vi "AlliGator Global Fit Decays.vi"(6 "IRF":cluster{"t Array":dbl[], "IRF Array":dbl[]}, 8 "error in (no error)":errorcluster, 10 "Abort Fit":refnum<vi>, 11 "Decay Graph":refnum<vi>) -> (0 "Error Out":errorcluster, 1 "Reduced Chi^2":dbl, 2 "R^2":dbl, 3 "Best Fit Parameters":dbl[](array[numeric]), 4 "Fit Output Message":string, 5 "Aborted?":bool)   [LabVIEW 2021, in "AlliGator Global Decay Fit.lvlib"]
uses:
  AlliGator Global Decay Fit.lvlib
  Settings/AlliGator Settings.lvlib
  Settings/AlliGator Settings List.ctl
  Fits/Decay Convolution/Decay Model.ctl
  Fits/Fits.lvlib
  Fits/Residual Type.ctl
  Fits/IRF(X)PSED/Decay Fit Parameters In List.ctl
  Decay Fit/AlliGator Decay Fit Parameter Constraints 2.ctl
  Decay Fit/AlliGator Decay Fit.lvlib
  Graphs/XY Graph/XY Graph Add-Ons.lvlib
  Fits/Global Fits/Global Fit Parameters Information.ctl
  Fits/Global Fits/Global Fit Data.ctl
  Time/Time.lvlib
  Fits/Abort Fit Global.vi
  Globals, Variables, Constants/AlliGator Globals, Variables & Constants.lvlib
  Globals, Variables, Constants/AlliGator Variables List.ctl
  Fits/Fit Calculation Method.ctl
  Fits/Non-linear Fitting Algorithm.ctl
  Fits/Non-linear Fitting Method v2.ctl
  Fits/Optimal Offset Selection Criterion.ctl
  Graphs/XY Graph/XY Graph Add Multiplots with Names v2.vi
  Graphs/LabVIEW Plot Interpolation.ctl
  Graphs/Graphs.lvlib
  Fits/IRF(X)PSED/Fit Weights Type v2.ctl
  Fits/IRF(X)PSED/Decay Fit Options v4.ctl
panel:
  # "see the License on the block diagram (Ctrl+E or Window:Show Block Diagram)"
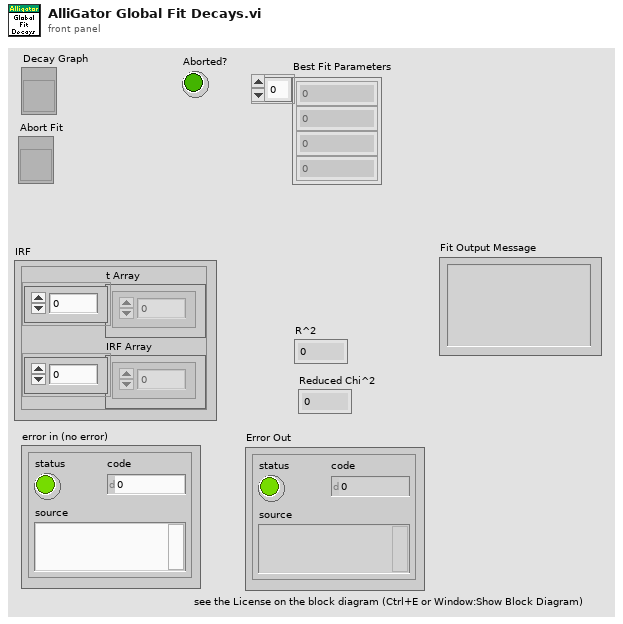
[diagram p1: front panel]
types:
  T1 = typedef "Fits.lvlib/Optimal Offset Selection Criterion.ctl" = enum16{"Min Chi^2", "Max R^2"}
  T2 = typedef "AlliGator Settings.lvlib/AlliGator Settings List.ctl" = enum16{"GUI:Visible Settings Tab", "GUI:Last Run Version", "Source Image:Use Image Histogram for Contrast", "Source Image:Low Count Pixels Rejection Options", "Source Image:High Count Pixels Rejection Options", "Source Image:Use Image Brightness", "Source Image:Blend Overlay with Image Background", "Source Image:Use Fixed ROI Diameter", "Source Image:ROI Diameter", "Source Image:ROI Center Color", "Source Image:Peak Threshold", "Source Image:Intensity Threshold", "Source Image:Image Binning Options", "Source Image:Image Smoothing Options", "Source Image:Image Histogram Active", "Source Image:Invert Binary Mask", "Source Image:Hot Pixel Removal", "Source Image:Overlay Analyzed ROI Center", "Source Image:Auto-Adjust Contrast", "Source Image:Histogram Lower Percentile", "Source Image:Histogram Upper Percentile", "Source Image:Save Source Image", "Source Image:Scale Bar Options", "Source Image:Image Resolution (Pixel Size)", "Source Image:Flatfield Correction", "Source Image:Show Dead Left Columns Correction", "Source Image:Dead Left Columns Correction", "Source Image:Image Pre-Processing Operations Order", "Source Image:Overlay ROI Median", "Source Image:Median Overlay Color", "Data Information:Gate Width", "Data Information:Nanotime Gate Separation", "Data Information:Macrotime Gate Separation", "Data Information:Gate Step", "Data Information:# Gates", "Data Information:Gate Image Exposure", "Data Information:Gate Image Integration", "Data Information:Gates to Skip", "Data Information:Gates to Keep", "Data Information:Define Gates to", "Data Information:Channel Name", "Data Information:Available Channel Names", "Data Information:Channel Arithmetic", "Data Information:Background File Subtraction", "Data Information:Background File", "Data Information:Background Scaling Factor", "Data Information:Background Pile-up Correction", "Data Information:Background Pixel Well Capacity", "Data Information:Laser Period", "Data Information:SYNC Period", "Data Information:Pile-up Correction", "Data Information:Pixel Well Capacity", "Data Information:Dataset Scaling Factor", "Fluorescence Decay_Decay Pre-Processing:Reverse Gates", "Fluorescence Decay_Decay Pre-Processing:Verbose Decay Pre-Processing", "Fluorescence Decay_Decay Pre-Processing:Use Decay Pre-Processing", "Fluorescence Decay_Decay Pre-Processing:Background Subtraction", "Fluorescence Decay_Decay Pre-Processing:Background Definition Range", "Fluorescence Decay_Decay Pre-Processing:Baseline Subtraction Method", "Fluorescence Decay_Decay Pre-Processing:Decay Pre-Processing Operations Order", "Fluorescence Decay_Decay Pre-Processing:Smoothing Parameter", "Fluorescence Decay_Decay Pre-Processing:Shift Decay", "Fluorescence Decay_Decay Pre-Processing:Decay Shift Parameters", "Fluorescence Decay_Decay Pre-Processing:Fold Decay", "Fluorescence Decay_Decay Pre-Processing:# Folds", "Fluorescence Decay_Decay Pre-Processing:1-Normalize Decay", "Fluorescence Decay_Decay Pre-Processing:[0-1]-Normalize Decay", "Fluorescence Decay_Decay Pre-Processing:Smoothen Decay", "Fluorescence Decay_Decay Pre-Processing:Extrapolate Decay", "Fluorescence Decay_Decay Pre-Processing:Use Periodicity", "Fluorescence Decay_Decay Pre-Processing:Use Cursors", "Fluorescence Decay_Decay Pre-Processing:Tail Fraction", "Fluorescence Decay_Decay Pre-Processing:Head Fraction", "Fluorescence Decay_Decay Pre-Processing:Additional Points", "Fluorescence Decay_Decay Pre-Processing:Straighten Decay", "Fluorescence Decay_Decay Pre-Processing:Constant Background", "Fluorescence Decay_Decay Pre-Processing:Pixel-Normalize Decay", "Fluorescence Decay_Advanced Analysis:Extract IRF instead of Decay", "Fluorescence Decay_Advanced Analysis:IRF Extraction Options", "Fluorescence Decay_Advanced Analysis:IRF Optimization Options", "Fluorescence Decay_Advanced Analysis:Square Pulse Options", "Fluorescence Decay_Advanced Analysis:IRF Order", "Fluorescence Decay_Advanced Analysis:IRF Time Constants", "Fluorescence Decay_Advanced Analysis:Wavelet Analysis Options", "Fluorescence Decay_Advanced Analysis:Average Lifetime Options", "Fluorescence Decay_Fit Options:Fit Options", "Fluorescence Decay_Fit Options:Use Legacy Fitting Approach", "Fluorescence Decay_Fit Options:Use Data Information Laser Period", "Fluorescence Decay_Fit Parameters:Displayed Fit Parameters", "Fluorescence Decay_Fit Parameters:Fit Parameter Constraints", "Fluorescence Decay_Fit Parameters:Export Tabulated Results", "Fluorescence Decay_Fit Parameters:MLE Baseline Offset Type", "Fluorescence Decay_Fit Parameters:MLE Baseline Offset", "Fluorescence Decay_Fit Parameters:Guess Parameter Names", "Fluorescence Decay_Fit Parameters:Guess Parameter Values", "Fluorescence Decay_Fit Parameters:Guess Parameters Options", "Fluorescence Decay_Fit Parameters:Optimal Offset Selection Criterion", "Fluorescence Decay_Styles:Show Last Decay Only", "Fluorescence Decay_Styles:Decay Graph Color Array", "Fluorescence Decay:Decay Graph Active", "Fluorescence Decay Statistics:Min Peak Value", "Fluorescence Decay Statistics:Reject Low Decay Peak Pixels", "Fluorescence Decay Statistics:Reject High Decay Peak Pixels", "Fluorescence Decay Statistics:Max Peak Value", "Time Traces:Use File Timestamp", "Time Traces:Time Step", "Time Traces:Use Intensity Correction File", "Time Traces:Intensity Correction File", "Phasor Plot:Phasor Plot Smoothing Options", "Phasor Plot:Phasor Plot Size", "Phasor Plot:Phasor Plot Graphics Options", "Phasor Plot:Cumulative Phasor Plot", "Phasor Plot:Use Phasor Brightness", "Phasor Plot:Blend Overlay with Phasor Background", "Phasor Plot:Save Phasor Plot", "Phasor Plot:Show References", "Phasor Plot:Phasor Ratio Decay Range", "Phasor Plot:Exponential Fading", "Phasor Plot:Phasor Ratio Reference Colors", "Phasor Plot:Reference Radius", "Phasor Plot:Show Color Map Vertices", "Phasor Plot:Phasor Plot Active", "Phasor Plot:Phasor Ratio Color Map Type", "Phasor Plot:Phasor Ratio Color Map", "Phasor Plot:Phasor Ratio Display Range", "Phasor Plot:Selected Image ROI(s)", "Phasor Plot:All Image ROIs", "Phasor Plot:Selected Phasor Plot ROI(s)", "Phasor Plot:All Phasor Plot ROIs", "Phasor Plot:Phasor Ratio Color-Coded Quantity", "Phasor Plot:Store Phasor Harmonics", "Phasor Plot:Draw Reference Segment", "Phasor Plot:User-Defined Quantity", "Phasor Plot:Color Scale High Color", "Phasor Plot:Color Scale Low Color", "Phasor Plot:Intensity-weighted Phasor Plot", "Phasor Graph:Phasor Frequency", "Phasor Graph:Phasor Ratio Type", "Phasor Graph:Pixel-level Phasor Computation", "Phasor Graph:Save Phasor Graph", "Phasor Graph:Phasor Graph Active", "Phasor Graph:Phasor SDV Options", "Phasor Graph:Intensity-weighted Phasor Graph", "Phasor Graph:Define Shortest Lifetime as", "Phasor Calibration:Use Backup Calibration if needed", "Phasor Calibration:Backup Calibration Type", "Phasor Calibration:Calibration Type", "Phasor Calibration:Calibration Lifetime", "Phasor Calibration:Calibration Map Algorithm", "Single-Exponential Phasor Locus (SEPL):Gate Parameters", "Single-Exponential Phasor Locus (SEPL):User-defined Gate", "Single-Exponential Phasor Locus (SEPL):User-defined IRF", "Single-Exponential Phasor Locus (SEPL):Phasor Parameters", "Single-Exponential Phasor Locus (SEPL):Decay & IRF Parameters", "Single-Exponential Phasor Locus (SEPL):Display Parameters", "Lifetime Analysis:Decay Analysis Parameters", "Lifetime Analysis:Lifetime Map Active", "Plugins:Python Settings", "Miscellaneous:Verbose Mode", "Miscellaneous:Beep after Script", "Miscellaneous:Saved Image File Format", "Miscellaneous:Exported Gate Image Settings", "Miscellaneous:Include Loading in Timing", "Miscellaneous:Verbose Settings Mode", "Miscellaneous:Histogram Options", "Miscellaneous:Beep on Error", "Miscellaneous:# Logical Processors Used", "Miscellaneous:ROI Description Max Characters", "Miscellaneous:Verbose Error Mode", "Miscellaneous:Transparent Mask Color"}
  T3 = typedef "Fits.lvlib/Decay Fit Options v4.ctl" = cluster{"Show Fit Residuals":bool, "Fit Model":T4, "Residual Type":T5, "Max Decay Percentile":dbl, "Min Decay Percentile":dbl, "Show Full Decay":bool, "Weights":T6, "Fitting Method":T7, "Compute Parameter Uncertainties":bool, "Periodic Boundaries":bool, "Model Calculation":T8, "Period":dbl[unit], "Termination Criteria":cluster{"Max Iterations":i32, "Max Function Calls":i32, "Max Time":dbl[unit], "Function Tolerance":dbl, "Parameter Tolerance":dbl, "Gradient Tolerance":dbl, "Min Lambda":dbl, "Max Lambda":dbl, "Initial Tick Count":u32}, "Offset Resolution":dbl[unit], "Use Local IRF":bool, "Fitting Algorithm":T9, "Show Confidence Interval ":bool, "Confidence Level":dbl}
  T4 = typedef "Fits.lvlib/Decay Model.ctl" = enum16{"1-Exponential", "2-Exponentials"}
  T5 = typedef "Fits.lvlib/Residual Type.ctl" = enum16{"Standard", "Normalized", "Reduced"}
  T6 = typedef "Fits.lvlib/Fit Weights Type v2.ctl" = enum16{"Unweighted", "1/Variance (Neyman)", "1/Variance (Pearson)", "Best of All"}
  T7 = typedef "Fits.lvlib/Non-linear Fitting Method v2.ctl" = enum16{"Least Square", "Least Absolute Residual", "Bisquare", "MLE", "-", "Best of All"}
  T8 = typedef "Fits.lvlib/Fit Calculation Method.ctl" = enum16{"Simulation", "Convolution", "Integration"}
  T9 = typedef "Fits.lvlib/Non-linear Fitting Algorithm.ctl" = enum16{"Levenberg-Marquardt", "Trust-Region Dogleg"}
  T10 = cluster{"Max Iterations":i32, "Max Function Calls":i32, "Max Time":dbl[unit], "Function Tolerance":dbl, "Parameter Tolerance":dbl, "Gradient Tolerance":dbl, "Min Lambda":dbl, "Max Lambda":dbl, "Initial Tick Count":u32}
  T11 = typedef "XY Graph Add-Ons.lvlib/XY Graph Refnum.ctl" = refnum<vi>
  T12 = typedef "AlliGator Globals, Variables & Constants.lvlib/AlliGator Variables List.ctl" = enum16{"---- GUI ----", "GUI:Initialization Status", "GUI:State Indicators Refnum", "GUI:Original AlliGator Menu Items", "GUI:Current Action Loop State", "GUI:Script in progress", "GUI:Playback", "GUI:Loop Playback", "GUI:Search ROI Used", "GUI:Search ROI", "Decay Graph Max Legend Size", "Intensity Graph Max Legend Size", "Decay Statistics Graph Max Legend Size", "Phasor Graph Max Legend Size", "Phasor Ratio Graph Max Legend Size", "Lifetime Graph Max Legend Size", "---- Files ----", "Files:Export Dataset Frames as Individual Files", "Files:Show Batch Export Help Balloons", "Files:Frames in Dataset", "Files:ptu File Frame Start Indices", "Files:Current Frame in Dataset", "Files:Current Frame Timestamp", "Files:Dataset Loaded", "Files:Dataset Metadata", "Files:Dataset Channel", "Files:Dataset Data Description", "Files:Background Dataset Metadata", "Files:Background Dataset Channel", "Files:Background Dataset Data Description", "Files:Background File Subtraction", "Files:Background File Path", "Files:Background File Pile-up Correction", "Files:Background File Pixel Well Capacity", "Files:Background File Scaling Factor", "Files:Current Dataset Load Settings", "Files:Dataset Path", "Files:ICCD-specific Information", "Files:Macrotime Gate Separation", "------ Python Plugins ------", "Python Plugins:Information", "Python Plugins:Python Session", "Python Plugins:Valid Python Session?", "---- Source Image ----", "Source Image:ROIs", "Source Image:Current ROI", "Source Image:ROI Event Refnum", "X_Source Image:Display Range", "X_Source Image:Palette Information", "X_Source Image:Type of Displayed Image", "X_Time Gate Slider", "Source Image:Palette List", "Source Image:Scale", "Source Image:ROI Overlay Color", "Source Image:Overlay to Erase", "Source Image:Is Displayed Image Accumulated", "Source Image:White Light Image Modified", "Source Image:Mask Image Modified", "---- Image Profile Window ----", "Image Profile:Window Event Refnum", "Image Profile:IntensityType", "Image Profile:Intensity Average Type", "Image Profile:Intensity-weighted SDV", "Image Profile:Box Profile Type", "Image Profile:Window Open", "Image Profile:Plotted Fit Parameter", "------ Phasor Graph -------", "Phasor Graph:Show Line", "---- Phasor Plot ---", "Phasor Plot:Parameters Changed", "Phasor Plot:FLI Dataset Modified since last Calculation", "Phasor Harmonics Data", "Selected Phasor Harmonics", "Phasor Harmonic Manager Event Refnum", "Phasor Plot:ROIs", "Phasor Plot:Current ROI", "Phasor Plot:ROI Event Refnum", "Phasor Plot:Image Reference Points", "Phasor Plot:Computed", "Phasor Plot:Palette Information", "Phasor Plot:Palette List", "Phasor Plot:Phasor Ratio Palette Information", "Phasor Plot:Phasor Ratio Palette List", "Phasor Plot:Image Scale", "Phasor Plot:Image Overlay to Erase", "Phasor Plot:Image Elements to Update", "Phasor Plot:Current Calculation Parameters", "Phasor Plot:Current Calibration Options", "Phasor Plot:Reset Cumulated Phasor Plot", "Phasor Plot:Reference 1", "Phasor Plot:Lifetime Reference 1", "Phasor Plot:Reference 1 Frequency", "Phasor Plot:Reference 2", "Phasor Plot:Lifetime Reference 2", "Phasor Plot:Reference 2 Frequency", "---- Decay Analysis ----", "Number of Selected Decays to Fit", "LS Fit Results", "LAR Fit Results", "BS Fit Results", "Last Decay Max - Min", "Best Fit Parameters", "Best Fit Parameter Names", "Actual Size X", "Actual Size Y", "Binning X", "Binning Y", "Actual # Gates", "Dataset Number", "Gates to...", "Gates Skipped", "Gates to keep", "Gate Step", "Gate Separation", "Reversed Gates", "Pile-up Correction", "Pixel Well Capacity", "Background Subtracted", "Background Subtraction Method", "Background Definition Range", "Background File (deprecated)", "Number of Dataset Accumulated", "Array of Accumulated Dataset Paths", "Do Averaged Datasets", "Destination File Path", "Process Plot Target", "Use 1/D as Phasor Frequency", "---- Decay Fit Parameter Map -----", "Decay Fit Parameter Map:Palette Information", "Decay Fit Parameter Map:Palette List", "Decay Fit Parameter Map:X Resolution", "Decay Fit Parameter Map:Y Resolution", "Decay Fit Parameter Map:Use Decay Fit Result Constraints", "Decay Fit Parameter Map:Decay Fit Result Constraints", "Decay Fit Parameter Map:Decay Fit Result Constraints Applied", "---- Parameter Map ----", "Parameter Map:Palette Information", "Parameter Map:Palette List", "------- Local Decay Window ---------", "Local Decay Graph Window:Event Refnum", "Local Decay Graph Window:Use normalized IRF for convolution", "----- Miscellaneous ----", "Misc:Skippable Dialog Windows Status"}
  T13 = typedef "AlliGator Decay Fit.lvlib/AlliGator Decay Fit Parameter Constraints 2.ctl" = cluster{"Fit Parameter":T14, "Min Value":dbl, "Max Value":dbl, "Global":bool, "Used":bool}
  T14 = typedef "Fits.lvlib/Decay Fit Parameters In List.ctl" = enum16{"Offset", "Baseline", "A_1", "tau_1", "A_2", "tau_2"}
  T15 = typedef "Fits.lvlib/Global Fit Data.ctl" = cluster{"Fit Data":variant, "Global Fit Parameter Information":T16, "# Points in Plots":i32[]}
  T16 = typedef "Fits.lvlib/Global Fit Parameters Information.ctl" = cluster{"Original Parameter Indices":i32[], "# Global Parameters":i32, "# Plot Specific Parameters":i32, "Global Parameter? Array":bool[]}
  T17 = typedef "Graphs.lvlib/LabVIEW Plot Interpolation.ctl" = enum16{"Point (.)", "Stepwise Right (--.)", "Line + Point (\\. /)", "Stepwise Left (.--)", "Stepwise Centered (-.-)", "Stepwise Vertical (|.|)", "Line (-)", "Use Previous Plot's Style"}
  T18 = cluster{"parameter minimum":dbl[], "parameter maximum":dbl[]}
  T19 = typedef "Fits.lvlib/Fit Plots.ctl" = cluster{"Fitted Decay":cluster{"t Array":dbl[], "Fitted Array":dbl[]}, "Residuals":cluster{"t Array":dbl[], "Residual Array":dbl[]}, "Upper CI Plot":cluster{"t Array":dbl[], "Residual Array":dbl[]}, "Lower CI Plot":cluster{"t Array":dbl[], "Residual Array":dbl[]}}
  T20 = typedef "Fits.lvlib/Non-linear Fit Output v4.ctl" = cluster{"best nonlinear fit":dbl[], "best fit parameters":dbl[], "R^2":dbl, "RMSE":dbl, "error out":errorcluster, "Fitting Method":T21, "number of function calls":i32, "number of iterations":i32, "covariance":T22, "Chi 2":dbl, "DOF":i32, "Fit Convergence Criterion":T23, "Fitting Algorithm":T9, "Weighted Fit":T6, "Gradient":dbl, "|Delta Chi 2|":dbl, "|Delta Chi 2|/Chi 2":dbl, "Max |Delta a| /|a|":dbl, "Lambda":dbl, "RSS":dbl, "AIC":dbl, "BIC":dbl, "Max number of function calls":i32, "Max number of iterations":i32, "IRF":T24, "IRF Normalization Factor":dbl, "Decay Normalization Factor":dbl, "Number of offset fits":i32, "Weighted Chi2":dbl, "Unweighted Chi2":dbl}
  T21 = typedef "Fits.lvlib/Nonlinear Fit Method.ctl" = enum16{"Least Square", "Least Absolute Residual", "Bisquare", "MLE"}
  T22 = typedef "NI_Matrix.lvlib/RealMatrix.ctl" = dbl[][]
  T23 = typedef "Fits.lvlib/Convergence Criteria.ctl" = enum16{"Continue", "Tolerances Exceeded", "Max Time Exceeded", "Max Iterations Exceeded", "Max Function Evaluations Exceeded", "Scale Range Exceeded"}
  T24 = typedef "XY Graph Add-Ons.lvlib/XY Graph Plot Data.ctl" = cluster{"X Array":dbl[], "Y Array":dbl[]}
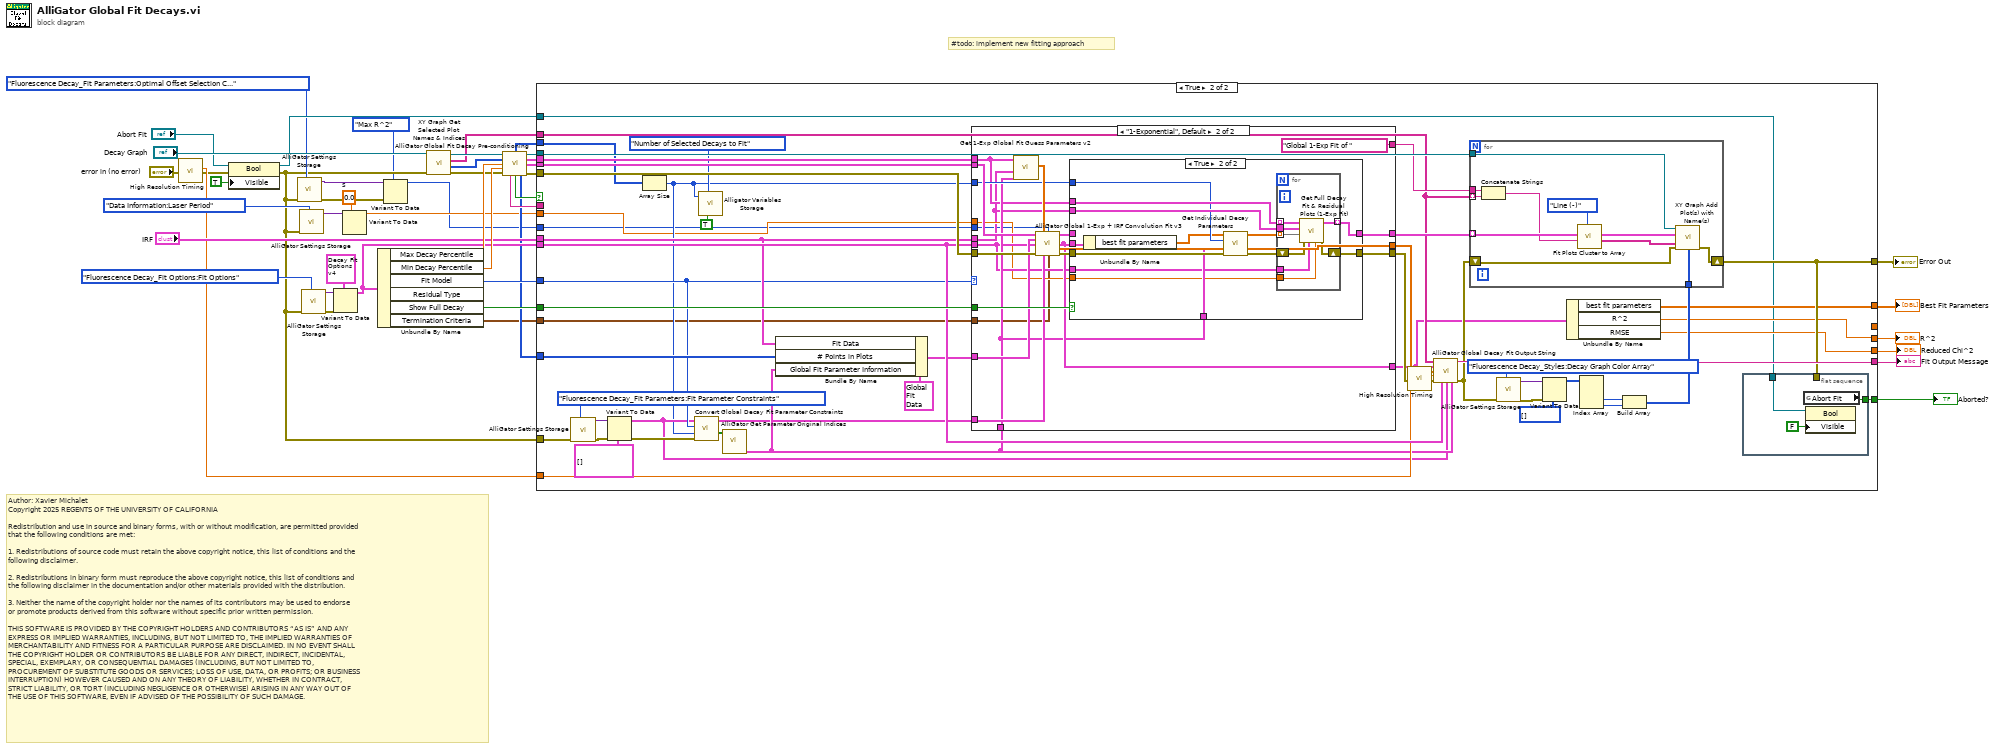
[diagram p0: block diagram]
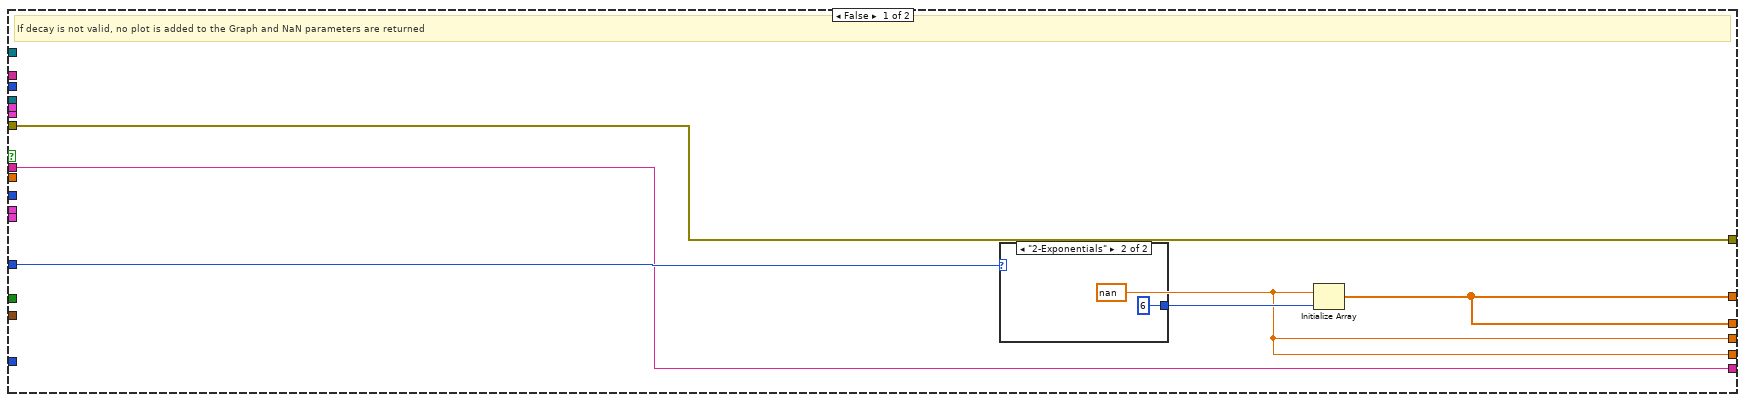
[diagram p2: hidden frame]
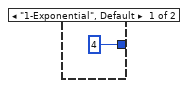
[diagram p3: hidden frame]
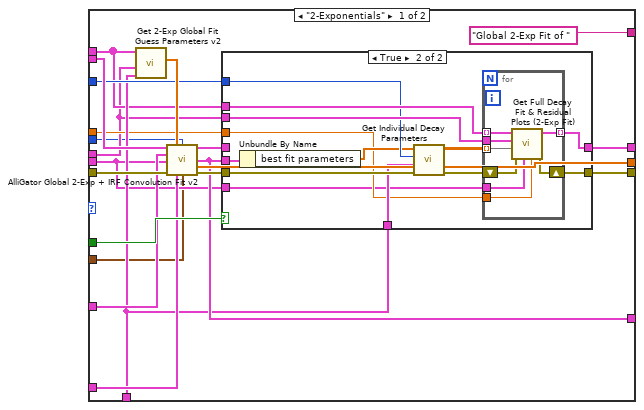
[diagram p4: hidden frame]
diagram:
  w13 = dbl[unit] 0.0  # s
  # "Author: Xavier Michalet\nCopyright 2025 REGENTS OF THE UNIVERSITY OF CALIFORNIA\n\nRedistribution and use in source and binary forms, with or without modification, are permitted provided\nthat the following conditions are met:\n\n1. Redistributions of source code must retain the above copyright notice, this list of conditions and the\nfollowing disclaimer.\n\n2. Redistributions in binary form must reproduce the above copyright notice, this list of conditions and\nthe following disclaimer in the documentation and/or other materials provided with the distribution.\n\n3. Neither the name of the copyright holder nor the names of its contributors may be used to endorse \nor promote products derived from this software without specific prior written permission.\n\nTHIS SOFTWARE IS PROVIDED BY THE COPYRIGHT HOLDERS AND CONTRIBUTORS “AS IS” AND ANY \nEXPRESS OR IMPLIED WARRANTIES, INCLUDING, BUT NOT LIMITED TO, THE IMPLIED WARRANTIES OF\nMERCHANTABILITY AND FITNESS FOR A PARTICULAR PURPOSE ARE DISCLAIMED. IN NO EVENT SHALL\nTHE COPYRIGHT HOLDER OR CONTRIBUTORS BE LIABLE FOR ANY DIRECT, INDIRECT, INCIDENTAL, \nSPECIAL, EXEMPLARY, OR CONSEQUENTIAL DAMAGES (INCLUDING, BUT NOT LIMITED TO, \nPROCUREMENT OF SUBSTITUTE GOODS OR SERVICES; LOSS OF USE, DATA, OR PROFITS; OR BUSINESS\nINTERRUPTION) HOWEVER CAUSED AND ON ANY THEORY OF LIABILITY, WHETHER IN CONTRACT, \nSTRICT LIABILITY, OR TORT (INCLUDING NEGLIGENCE OR OTHERWISE) ARISING IN ANY WAY OUT OF\nTHE USE OF THIS SOFTWARE, EVEN IF ADVISED OF THE POSSIBILITY OF SUCH DAMAGE."
  # "#todo: implement new fitting approach"
  n1 = call "High Resolution Timing.vi"("Error In"="error in (no error)") -> ("elapsed (relative) seconds"=w21:dbl, "Error Out"=w9:errorcluster)  [unwired: 16 in, 1 out]
  n2 = property class="Bool"(reference="Abort Fit", error in=w9, "Visible"=TRUE) -> (reference out=w8:refnum<vi>, error out=w5:errorcluster)
  n3 = call "AlliGator Settings Storage.vi"("AlliGator Settings List"=AlliGator_Settings_List."Fluorescence Decay_Fit Parameters:Optimal Offset Selection Criterion", "Error In"=w5) -> ("Error Out"=w4:errorcluster, "Variant Data out"=w3:variant)  [unwired: 8 in]
  n4 = call "AlliGator Settings Storage.vi"("AlliGator Settings List"=AlliGator_Settings_List."Data Information:Laser Period", "Error In"=w5) -> ("Variant Data out"=w14:variant)  [unwired: 8 in, 1 out]
  n5 = call "AlliGator Settings Storage.vi"("AlliGator Settings List"=AlliGator_Settings_List."Fluorescence Decay_Fit Options:Fit Options", "Error In"=w5) -> ("Error Out"=w41:errorcluster, "Variant Data out"=w42:variant)  [unwired: 8 in]
  n6 = Variant To Data(error in=w41, type=T3 {"Show Fit Residuals"=TRUE, "Fit Model"=enum."1-Exponential", "Residual Type"=enum."Standard", "Max Decay Percentile"=0.0, "Min Decay Percentile"=0.0, "Show Full Decay"=TRUE, "Weights"=enum."Unweighted", "Fitting Method"=enum."Least Square", "Compute Parameter Uncertainties"=TRUE, "Periodic Boundaries"=TRUE, "Model Calculation"=enum."Simulation", "Period"=1.2500000000000001e-08, "Termination Criteria"={"Max Iterations"=1000, "Max Function Calls"=0, "Max Time"=1000.0, "Function Tolerance"=1e-06, "Parameter Tolerance"=1e-06, "Gradient Tolerance"=0.0, "Min Lambda"=1e-06, "Max Lambda"=1e-06, "Initial Tick Count"=0}, "Offset Resolution"=1.2500000000000001e-08, "Use Local IRF"=TRUE, "Fitting Algorithm"=enum."Levenberg-Marquardt", "Show Confidence Interval "=TRUE, "Confidence Level"=95.0} ("Fit Options"), Variant=w42) -> (data=w32:T3)  [unwired: 1 out]
  n7 = Variant To Data(type=w13, Variant=w14) -> (data=w12:dbl[unit])  [unwired: 1 in, 1 out]
  n8 = Unbundle By Name(w32) -> ("Max Decay Percentile"=w36:dbl, "Min Decay Percentile"=w35:dbl, "Fit Model"=w31:T4, "Show Full Decay"=w34:bool, "Termination Criteria"=w11:T10)  [unwired: 1 out]
  n9 = Variant To Data(error in=w4, type=Optimal_Offset_Selection_Criterion."Max R^2" ("Optimal Offset Selection Criterion"), Variant=w3) -> (data=w1:T1)  [unwired: 1 out]
  n10 = call "XY Graph Get Selected Plot Names & Indices.vi"("error in (no error)"=w5, "XY Graph in"="Decay Graph") -> ("error out"=w17:errorcluster, "Selected Plot Indices"=w16:i32[], "Selected Plot Names"=w24:string[], "XY Graph out"=w29:T11)  [unwired: 5 in, 1 out]
  n11 = call "AlliGator Global Fit Decay Pre-conditioning.vi"("XYGraph in"=w29, "Selected Plots"=w16, "Max Decay Percentile (1)"=w36, "Min Decay Percentile (0)"=w35, "error in (no error)"=w17) -> ("Index Max Array"=w25:i32[], "XYGraph out"=w46:refnum<vi>, "Full Decays"=w23:cluster{"t Array":dbl[], "Value Array":dbl[]}[], "Clipped Decays"=w27:cluster{"t Array":dbl[], "Value Array":dbl[]}[], "Message"=w28:string, "Is Valid?"=w33:bool, "# Points"=w18:i32[], "error out"=w19:errorcluster)  [unwired: 1 in, 2 out]
  n12 = case shown="True" w33 {
    tunnel: w46 -> [_ w107]
    tunnel: [w52 w90] -> w45
    tunnel: [w47 w105] -> w44
    tunnel: [w49 w61] -> w39
    tunnel: [w49 _] -> _
    tunnel: [w48 w60] -> w38
    tunnel: w31 -> [w51 w84]
    tunnel: [w48 w59] -> w37
    tunnel: "IRF" -> [_ w88]
    tunnel: w34 -> [_ w101]
    tunnel: w19 -> [w52 w100]
    tunnel: w32 -> [_ w98]
    tunnel: w28 -> [w47 _]
    tunnel: w27 -> [_ w97]
    tunnel: w25 -> [_ w64]
    tunnel: w24 -> [_ w95]
    tunnel: w23 -> [_ w96]
    tunnel: w21 -> [_ w93]
    tunnel: [_ w91] -> w20
    tunnel: w18 -> [_ w87]
    tunnel: w5 -> [_ w78]
    tunnel: w12 -> [_ w58]
    tunnel: w11 -> [_ w57]
    tunnel: w8 -> [_ w56]
    tunnel: w1 -> [_ w55]
    frame False {
      w48 = nan ("element")
      # "If decay is not valid, no plot is added to the Graph and NaN parameters are returned"
      n13 = case shown="\"2-Exponentials\"" w51 {
        tunnel: [4 ("dimension size") 6 ("dimension size")] -> w50
        frame "1-Exponential", Default {
        }
        frame "2-Exponentials" {
        }
      }
      n14 = Initialize Array(w48, w50) -> (w49:dbl[])
    }
    frame True {
      n15 = call "AlliGator Settings Storage.vi"("AlliGator Settings List"=AlliGator_Settings_List."Fluorescence Decay_Fit Parameters:Fit Parameter Constraints", "Error In"=w78) -> ("Error Out"=w80:errorcluster, "Variant Data out"=w81:variant)  [unwired: 8 in]
      n16 = Variant To Data(error in=w80, type=T13[] [] ("Fit Parameter Constraints"), Variant=w81) -> (data=w75:T13[], error out=w76:errorcluster)
      n17 = Array Size(array=w64) -> (size(s)=w63:i32)
      n18 = call "Convert Global Decay Fit Parameter Constraints.vi"("Error In"=w76, "# Plots"=w63, "Fit Model"=w84, "Fit Parameter Constraints"=w75) -> ("Global Parameters?"=w83:bool[], "Parameter Bounds"=w82:T18)  [unwired: 5 in, 1 out]
      n19 = call "Alligator Variables Storage.vi"("Get(F)/Set"=TRUE, "AlliGator Variable"=AlliGator_Variables_List."Number of Selected Decays to Fit" ("Alligator Variable"), "Data in"=w63) -> ()  [unwired: 6 in, 3 out]
      n20 = call "AlliGator Get Parameter Original Indices.vi"("Parameter Types"=w83) -> ("Global Fit Parameter Info"=w85:T16)  [unwired: 8 in, 2 out]
      n21 = Bundle By Name(cluster=T15 {"Fit Data"=variant(cluster{"t Array":dbl[], "IRF Array":dbl[]} {"t Array"=[], "IRF Array"=[]}), "Global Fit Parameter Information"={"Original Parameter Indices"=[], "# Global Parameters"=0, "# Plot Specific Parameters"=0, "Global Parameter? Array"=[]}, "# Points in Plots"=[]} ("Global Fit Data"), "Fit Data"=w88, "# Points in Plots"=w87, "Global Fit Parameter Information"=w85) -> (w86:T15)
      n22 = case shown="\"1-Exponential\", Default" w84 {
        tunnel: w88 -> [w124 w168]
        tunnel: w100 -> [w142 w186]
        tunnel: ["Global 2-Exp Fit of " ("string") "Global 1-Exp Fit of " ("string")] -> w106
        tunnel: [w138 w181] -> w99
        tunnel: [w140 w184] -> w103
        tunnel: [w122 w182] -> w104
        tunnel: w101 -> [w139 w183]
        tunnel: w98 -> [w127 w172]
        tunnel: w82 -> [w137 w180]
        tunnel: w97 -> [w134 w178]
        tunnel: w86 -> [w132 w176]
        tunnel: w85 -> [w129 w173]
        tunnel: w96 -> [w126 w170]
        tunnel: w63 -> [w131 w175]
        tunnel: [w130 w174] -> w62
        tunnel: w58 -> [w128 w171]
        tunnel: w57 -> [w125 w169]
        tunnel: w55 -> [w123 w167]
        frame "2-Exponentials" {
          n23 = call "Get 2-Exp Global Fit Guess Parameters v2.vi"("Global Fit Parameter Info"=w129, "IRF"=w124, "Full Decays"=w126) -> ("Initial Parameters"=w133:dbl[])  [unwired: 8 in]
          n24 = call "AlliGator Global 2-Exp + IRF Convolution Fit v2.vi"("Decays"=w134, "Initial Parameters"=w133, "Optimal Offset Selection Criterion"=w123, "Global Fit Parameters Info"=w132, "Fit Options"=w127, "error in (no error)"=w142, "parameter bounds"=w137, "Termination Criteria"=w125) -> ("Fit Plots Array"=w136:T19[], "Fit Output"=w130:T20, "Delta Best Fit Parameters"=w140:dbl[], "error out"=w135:errorcluster)  [unwired: 4 in]
          n25 = case shown="True" w139 {
            tunnel: w136 -> [w143 _]
            tunnel: w135 -> [w144 w155]
            tunnel: [w144 w157] -> w138
            tunnel: w124 -> [_ w156]
            tunnel: w129 -> [_ w154]
            tunnel: w126 -> [_ w152]
            tunnel: w131 -> [_ w150]
            tunnel: w130 -> [_ w149]
            tunnel: w128 -> [_ w147]
            tunnel: w127 -> [_ w146]
            tunnel: [w143 w145] -> w122
            frame False {
            }
            frame True {
              n26 = Unbundle By Name(w149) -> ("best fit parameters"=w148:dbl[])
              n27 = call "Get Individual Decay Parameters.vi"("Error In"=w155, "Global Fit Parameter Info"=w154, "# Decays"=w150, "Global Fit Parameters Array"=w148) -> ("Error Out"=w151:errorcluster, "All Parameters Array"=w153:dbl[][])  [unwired: 4 in, 2 out]
              n28 = for {
                tunnel: w156 -> [w165]
                tunnel: w153 -> [w164] mode=indexing
                tunnel: w152 -> [w163] mode=indexing
                shift-right: [w161] -> w157
                shift-left: w151 -> [w162]
                tunnel: [w160] -> w145 mode=indexing
                tunnel: w147 -> [w159]
                tunnel: w146 -> [w158]
                n29 = call "Get Full Decay Fit & Residual Plots (2-Exp Fit).vi"("Laser Period"=w159, "Fit Options"=w158, "Error In"=w162, "Best Fit Parameters"=w164, "IRF"=w165, "Full Decay"=w163) -> ("Error Out"=w161:errorcluster, "Fit Plots"=w160:T19)  [unwired: 4 in]
              }
            }
          }
        }
        frame "1-Exponential", Default {
          n30 = call "Get 1-Exp Global Fit Guess Parameters v2.vi"("Global Fit Parameter Info"=w173, "IRF"=w168, "Full Decays"=w170) -> ("Initial Parameters"=w177:dbl[])  [unwired: 8 in]
          n31 = call "AlliGator Global 1-Exp + IRF Convolution Fit v3.vi"("Decays"=w178, "Initial Parameters"=w177, "Optimal Offset Selection Criterion"=w167, "Global Fit Parameters Info"=w176, "Fit Options"=w172, "error in (no error)"=w186, "parameter bounds"=w180, "Termination Criteria"=w169) -> ("Fit Plots Array"=w166:T19[], "Fit Output"=w174:T20, "Delta Best Fit Parameters"=w184:dbl[], "error out"=w179:errorcluster)  [unwired: 4 in]
          n32 = case shown="True" w183 {
            tunnel: [w187 w194] -> w182
            tunnel: w179 -> [w188 w199]
            tunnel: [w188 w201] -> w181
            tunnel: w168 -> [_ w200]
            tunnel: w173 -> [_ w198]
            tunnel: w170 -> [_ w196]
            tunnel: w175 -> [_ w193]
            tunnel: w174 -> [_ w192]
            tunnel: w172 -> [_ w190]
            tunnel: w171 -> [_ w189]
            tunnel: w166 -> [w187 _]
            frame False {
            }
            frame True {
              n33 = Unbundle By Name(w192) -> ("best fit parameters"=w191:dbl[])
              n34 = call "Get Individual Decay Parameters.vi"("Error In"=w199, "Global Fit Parameter Info"=w198, "# Decays"=w193, "Global Fit Parameters Array"=w191) -> ("Error Out"=w195:errorcluster, "All Parameters Array"=w197:dbl[][])  [unwired: 4 in, 2 out]
              n35 = for {
                tunnel: w200 -> [w209]
                tunnel: w197 -> [w208] mode=indexing
                tunnel: w196 -> [w207] mode=indexing
                shift-right: [w205] -> w201
                shift-left: w195 -> [w206]
                tunnel: [w204] -> w194 mode=indexing
                tunnel: w190 -> [w203]
                tunnel: w189 -> [w202]
                n36 = call "Get Full Decay Fit & Residual Plots (1-Exp Fit).vi"("Laser Period"=w202, "Fit Options"=w203, "Error In"=w206, "Best Fit Parameters (All)"=w208, "IRF"=w209, "Full Decay"=w207) -> ("Error Out"=w205:errorcluster, "Fit Plots"=w204:T19)  [unwired: 4 in]
              }
            }
          }
        }
      }
      n37 = call "High Resolution Timing.vi"("relative seconds (NaN)"=w93, "Error In"=w99) -> ("elapsed (relative) seconds"=w92:dbl, "Error Out"=w94:errorcluster)  [unwired: 15 in, 1 out]
      n38 = call "AlliGator Global Decay Fit Output String.vi"("Plot Names"=w95, "Fit Output"=w62, "Delta Best Fit Parameters"=w103, "elapsed (relative) seconds"=w92, "Error In"=w94, "Fit Options"=w98, "Fit Parameter Constraints"=w75, "Global Fit Parameter Info"=w85) -> ("Fit Output Message"=w105:string, "Error Out"=w67:errorcluster)  [unwired: 6 in]
      n39 = call "AlliGator Settings Storage.vi"("AlliGator Settings List"=AlliGator_Settings_List."Fluorescence Decay_Styles:Decay Graph Color Array", "Error In"=w67) -> ("Error Out"=w73:errorcluster, "Variant Data out"=w72:variant)  [unwired: 8 in]
      n40 = Variant To Data(error in=w73, type=u32[] [] ("appended array"), Variant=w72) -> (data=w74:u32[])  [unwired: 1 out]
      n41 = Unbundle By Name(w62) -> ("best fit parameters"=w61:dbl[], "R^2"=w60:dbl, "RMSE"=w59:dbl)
      n42 = Index Array(array=w74) -> (element #2=w69:u32, element #3=w68:u32)  [unwired: 3 in, 1 out]
      n43 = Build Array(w69, w68) -> (w102:u32[])
      n44 = for {
        tunnel: w107 -> [w119]
        tunnel: w106 -> [w121]
        tunnel: w104 -> [w115] mode=indexing
        tunnel: w102 -> [w116]
        shift-right: [w117] -> w90
        shift-left: w67 -> [w118]
        tunnel: w95 -> [w120] mode=indexing
        n45 = Concatenate Strings(w121, w120) -> (w114:string)
        n46 = call "Fit Plots Cluster to Array.vi"("Plot Interpolation"=LabVIEW_Plot_Interpolation."Line (-)", "Decay Fit Plot Name"=w114, "Fit Plots in"=w115) -> ("Plot Names"=w113:string[], "Fit Plot Array"=w112:cluster{"t Array":dbl[], "Fitted Array":dbl[]}[])  [unwired: 6 in, 1 out]
        n47 = call-poly "XY Graph Add Plot(s) with Name(s).vi"("XYGraph in"=w119, "Array of Plots"=w112, "Array of Plot Names (\"Plot\")"=w113, "error in (no error)"=w118, "Plot Colors (Default)"=w116) -> ("error out"=w117:errorcluster)  [unwired: 6 in, 4 out]
      }
      n48 = flat-sequence {
        tunnel: [w110] -> w91
        tunnel: w90 -> [_]
        tunnel: w56 -> [w108]
        frame #0 {
          n49 = global read "Abort Fit Global.vi" "Abort Fit"() -> (w110:bool)
          n50 = property class="Bool"(reference=w108, "Visible"=FALSE) -> ()  [unwired: 1 in, 2 out]
        }
      }
    }
  }
  "Error Out" <- w45
  "Fit Output Message" <- w44
  "Best Fit Parameters" <- w39
  "R^2" <- w38
  "Reduced Chi^2" <- w37
  "Aborted?" <- w20
